vi "Page_Source_Initialize.vi"(8 "error in (no error)":errorcluster, 9 "ctlReferences":T1, 11 "AB_EXE in":refnum<class "AB_EXE.lvclass">) -> (0 "error out":errorcluster, 1 "supportedFunctions":T2, 3 "AB_EXE out":refnum<class "AB_EXE.lvclass">)   [LabVIEW 2020, in "AB_EXE.lvclass"]
uses:
  <vilib>/AppBuilder/AB_Classes/EXE/AB_EXE.lvclass
  <resource>/Framework/Providers/Builds/AppBuilder/AB_UI_Page_Source_Files_supportedFunctions.ctl
  <vilib>/AppBuilder/AB_Source_Inclusion.ctl
  <resource>/Framework/Providers/Builds/AppBuilder/AB_UI_Page_Source_Files_References.ctl
  <vilib>/AppBuilder/AB_Classes/Application/AB_Application.lvclass
  <vilib>/AppBuilder/AB_Classes/EXE/common/AB_EXE.lvlib
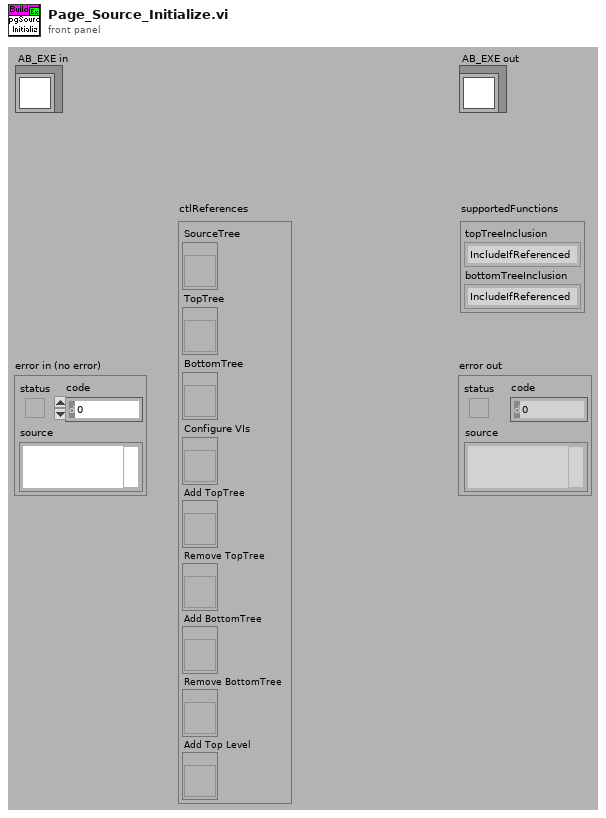
[diagram p1: front panel]
types:
  T1 = typedef "AB_UI_Page_Source_Files_References.ctl" = cluster{"SourceTree":refnum<vi>, "TopTree":refnum<vi>, "BottomTree":refnum<vi>, "Configure VIs":refnum<vi>, "Add TopTree":refnum<vi>, "Remove TopTree":refnum<vi>, "Add BottomTree":refnum<vi>, "Remove BottomTree":refnum<vi>, "Add Top Level":refnum<vi>}
  T2 = typedef "AB_UI_Page_Source_Files_supportedFunctions.ctl" = cluster{"topTreeInclusion":T3, "bottomTreeInclusion":T3}
  T3 = typedef "AB_Source_Inclusion.ctl" = enum16{"IncludeIfReferenced", "Include", "Exclude", "TopLevel"}
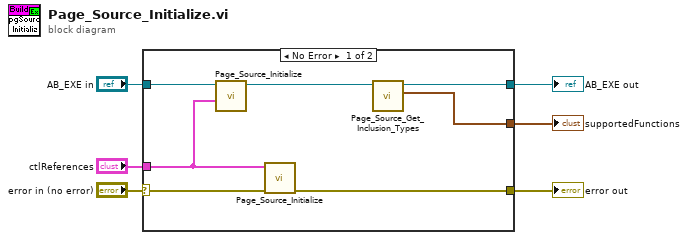
[diagram p0: block diagram]
diagram:
  n1 = case shown="No Error" "error in (no error)" {
    selector: "error in (no error)" -> [w8 w15]
    tunnel: [w7 w15] -> w2
    tunnel: "AB_EXE in" -> [w11 w14]
    tunnel: "ctlReferences" -> [w9 _]
    tunnel: [w12 _] -> w3
    tunnel: [w13 w14] -> w1
    frame No Error {
      n2 = call-parent <vilib>:"Page_Source_Initialize.vi"("ctlReferences"=w9, "AB_Build in"=w11) -> ("AB_Build out"=w10:refnum<class "AB_EXE.lvclass">)  [unwired: 7 in, 2 out]
      n3 = call <vilib>:"Page_Source_Initialize.vi"("error in (no error)"=w8, "ctlReferences"=w9) -> ("error out"=w7:errorcluster)  [unwired: 9 in]
      n4 = call-dynamic "Page_Source_Get_Inclusion_Types.vi"("AB_EXE in"=w10) -> ("supportedFunctions"=w12:T2, "AB_EXE out"=w13:refnum<class "AB_EXE.lvclass">)  [unwired: 8 in, 1 out]
    }
    frame Error {
    }
  }
  "error out" <- w2
  "supportedFunctions" <- w3
  "AB_EXE out" <- w1
